vi "main.vi"() -> ()   [LabVIEW 2020]
uses:
  Desktop/eTPC/subVIs for MKS/INITIALIZATION PFEIFFER.ctl
  INITIALIZATION.ctl
  <instrlib>/PV ActiveLine/Public/Action-Status/PV ActiveLine - Sensor On-Off (TPG362).vi
  <instrlib>/PV ActiveLine/Public/Data/PV ActiveLine - Measurement Data all Gauges (TPG362).vi
  <instrlib>/PV ActiveLine/PV ActiveLine.lvlib
panel:
  in  "BACK TO CONFIG":bool
  out "CAEN":string
  out "NI DAQ":string
  out "PF":string
  out "MKS":string
  out "PF UNIT":i8 min=0 max=2
  out "PF UNIT":i8 min=0 max=2
  out "NI RELAYS STATUS":bool[](array[boolean]) caption="data"
  out "PF RESAYS STATUS":bool[](array[boolean])
  out "MKS RELAYS STATUS":bool[](array[boolean])
  out "MKS FLOW":dbl[](array[numeric])
  in  "NI OPEN VALVE":bool
  out "PF 4":bool
  out "PF 3":bool
  out "PF 2":bool
  out "PF 1":bool
  out "MKS 12":bool
  out "MKS 11":bool
  out "MKS 10":bool
  out "MKS 9":bool
  out "MKS 8":bool
  out "MKS 7":bool
  out "MKS 6":bool
  out "MKS 5":bool
  out "MKS 4":bool
  out "MKS 3":bool
  out "MKS 2":bool
  out "MKS1":bool
  out "NI 8":bool
  out "NI 7":bool
  out "NI 6":bool
  out "ALARM":bool
  out "V4":bool
  out "V3":bool
  out "V2":bool
  out "V1":bool
  in  "Tab Control":enum32{"MKS", "PFEIFEER", "CAEN", "DAQ", "LOG"}(tab)
  in  "CONNECT WITH MKS":bool
  in  "MKS":T1={"ADDRESS"="001", "BAUDE RATE"=19200, "VISA RESOURCE NAME"="", "parity (0:none)"=0} caption="Cluster 2" {"parity (0:none)" items=["None", "Odd", "Even", "Mark", "Space"]; "BAUDE RATE" items=["38400"=38400, "19200"=19200, "9600"=9600, "4800"=4800]}
  in  "MKS SET UNIT":string(combo)="MBAR" caption="MKS UNITS"
  in  "CONNECT WITH PFIFER":bool
  in  "PFEIFFER":T2={"BAUDE RATE"=enum."9600", "VISA RESOURCE NAME"=""}
  out "Device Type":string
  out "Serial Number":string
  out "Gauge out":string[](array[string])
  in  "PF SET UNIT":i8(ring) items=["mbar / bar", "Torr", "Pascal", "Micron", "hPascal (default)", "Volt"]
  in  "CONNECT WITH CAEN":bool
  in  "CAEN 2":T2={"BAUDE RATE"=enum."9600", "VISA RESOURCE NAME"=""}
  out "CAEN MODEL":string
  in  "DAQ NAME":tag="Dev3"
  in  "CONNECT WITH DAQ":bool
  in  "LOG FILE":path
  out "FILE":string
  out "status":bool
  out "code":i32
  out "FILENAME":refnum<file>
  in  "CAEN SET VOLTAGE B":bool
  in  "CAEN SET CURRENT B":bool
  out "PF Pressure CH1":dbl format="%.3e"
  out "PF Pressure CH2":dbl format="%.3e"
  out "CAEN MON CURRENT":dbl[](array[numeric])
  out "CAEN MON VOLTAGE":dbl[](array[numeric])
  in  "CAEN SET VOLTAGE":dbl
  in  "CAEN SET CURRENT":dbl
  in  "CAEN CHANNEL":string(combo)
  out "MKS PRESSURE":dbl[](array[numeric])
  out "MON ERROR":errorcluster
  in  "START":bool
  out "MKS UNIT":string
  out "INITN ERROR":errorcluster
  out "END ERROR":errorcluster
  in  "stop":bool
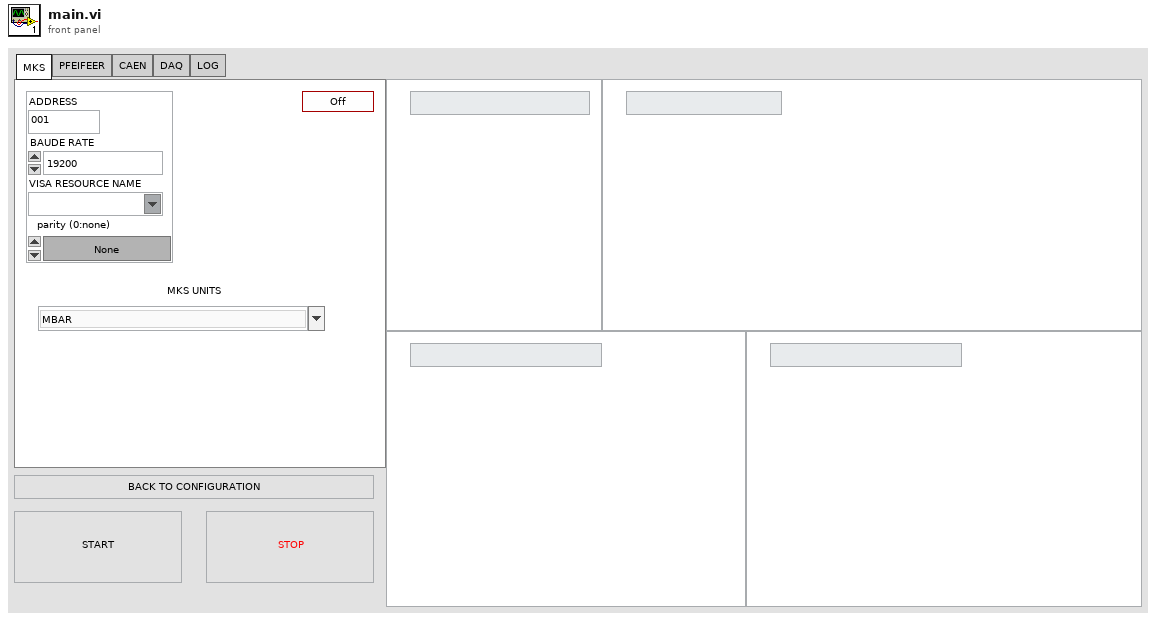
[diagram p1: front panel]
types:
  T1 = typedef "INITIALIZATION.ctl" = cluster{"ADDRESS":string, "BAUDE RATE":u32, "VISA RESOURCE NAME":refnum<visa-resource-name>, "parity (0:none)":u16}
  T2 = typedef "INITIALIZATION PFEIFFER.ctl" = cluster{"BAUDE RATE":enum32{"38400", "19200", "9600", "4800"}, "VISA RESOURCE NAME":refnum<visa-resource-name>}
  T3 = enum16{"open", "replace", "create", "open or create", "replace or create", "replace or create with confirmation"}
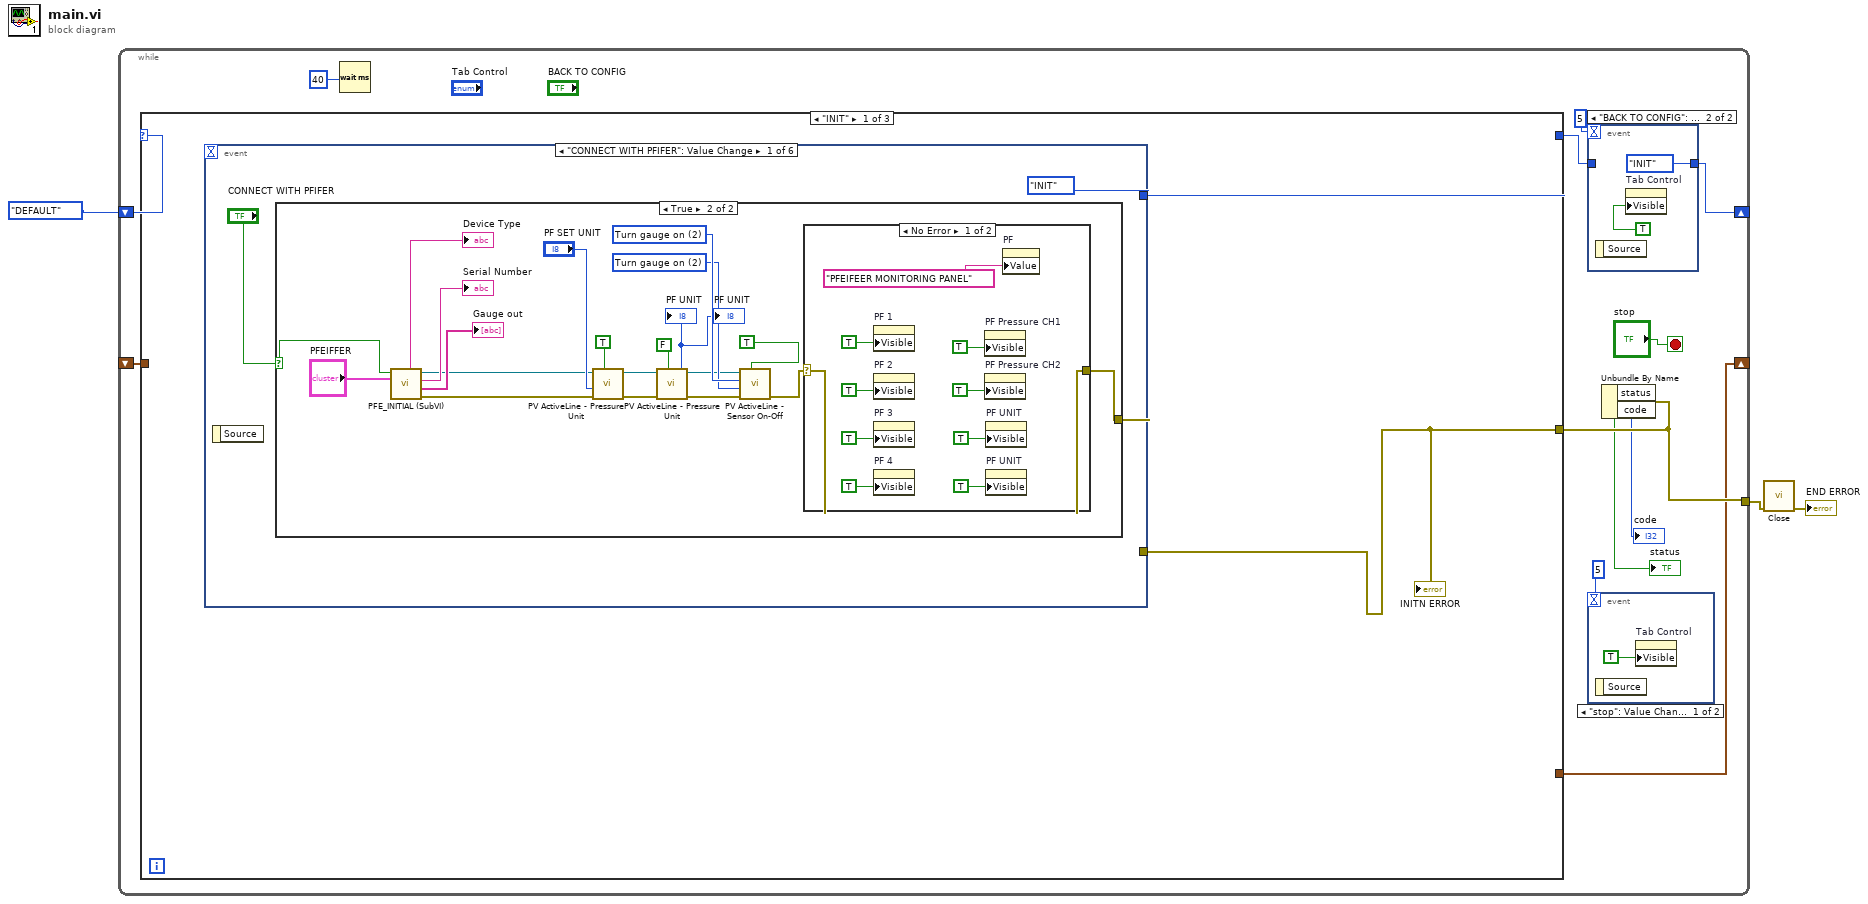
[diagram p0: block diagram]
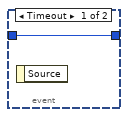
[diagram p2: hidden frame]
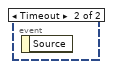
[diagram p3: hidden frame]
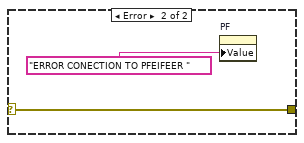
[diagram p5: hidden frame]
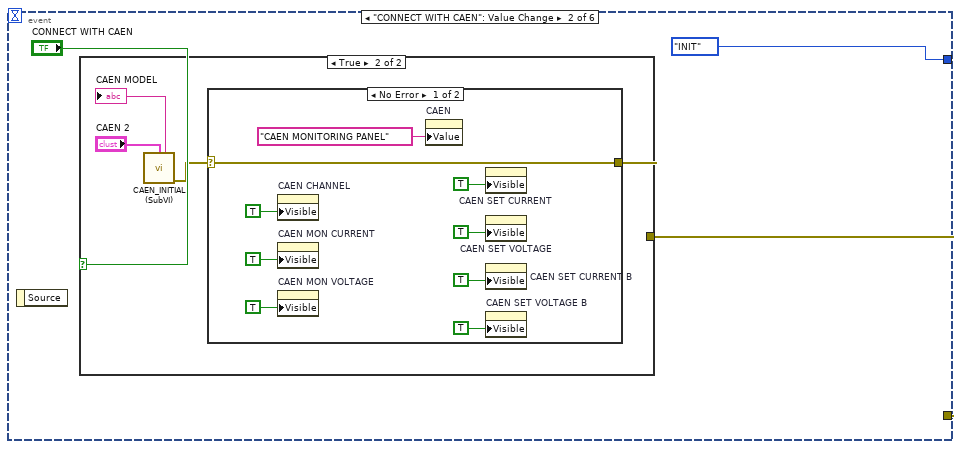
[diagram p6: hidden frame]
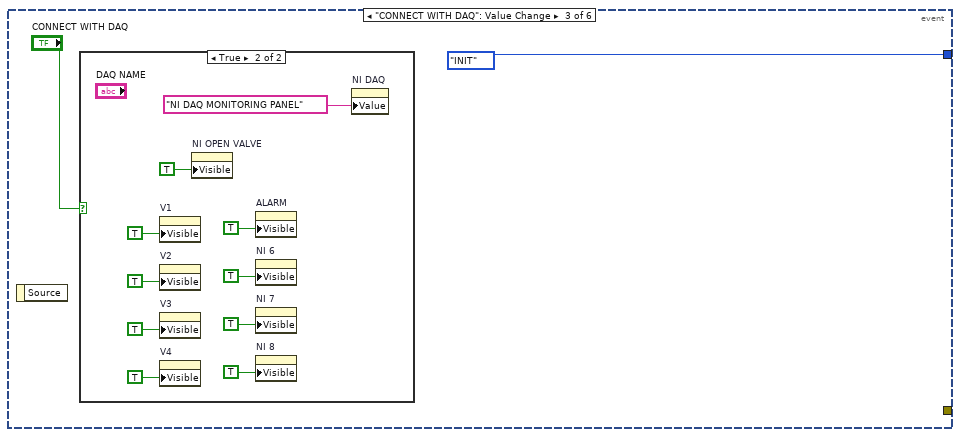
[diagram p9: hidden frame]
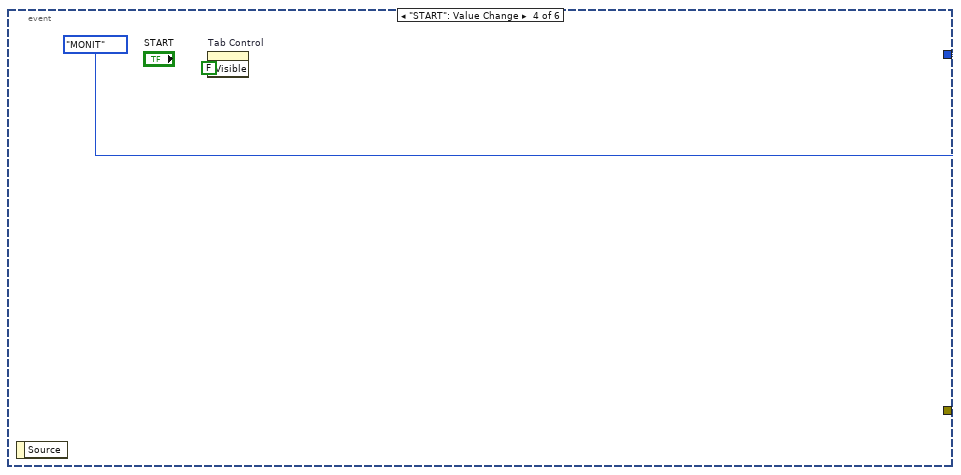
[diagram p11: hidden frame]
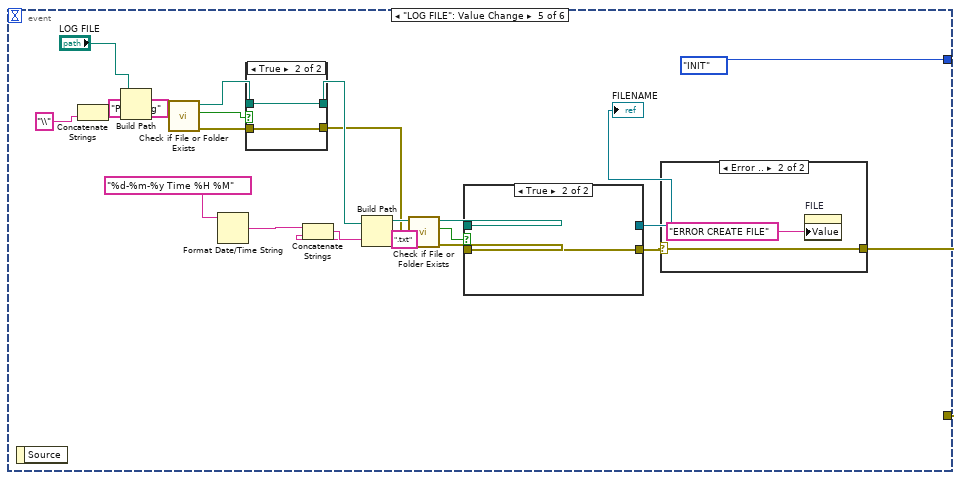
[diagram p12: hidden frame]
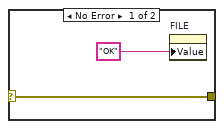
[diagram p13: hidden frame]
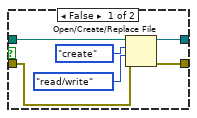
[diagram p14: hidden frame]
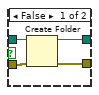
[diagram p15: hidden frame]
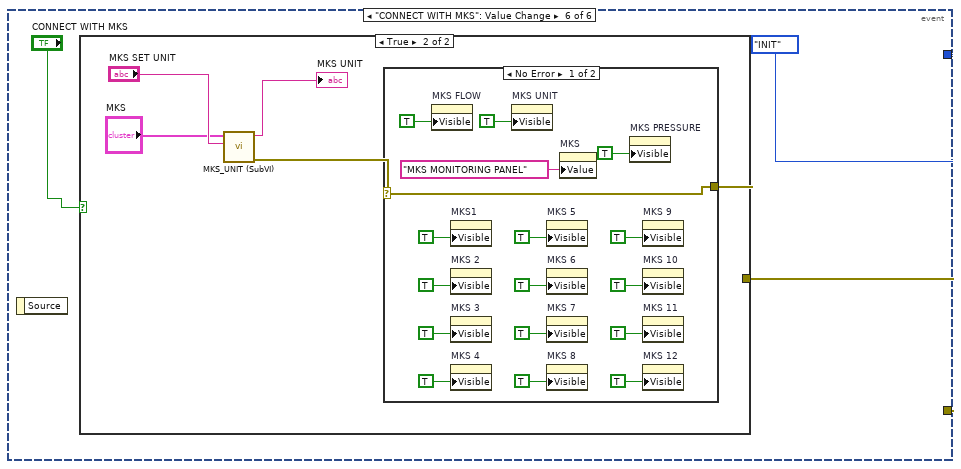
[diagram p16: hidden frame]
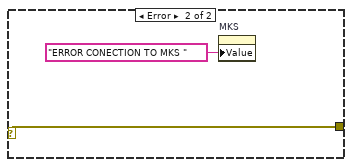
[diagram p18: hidden frame]
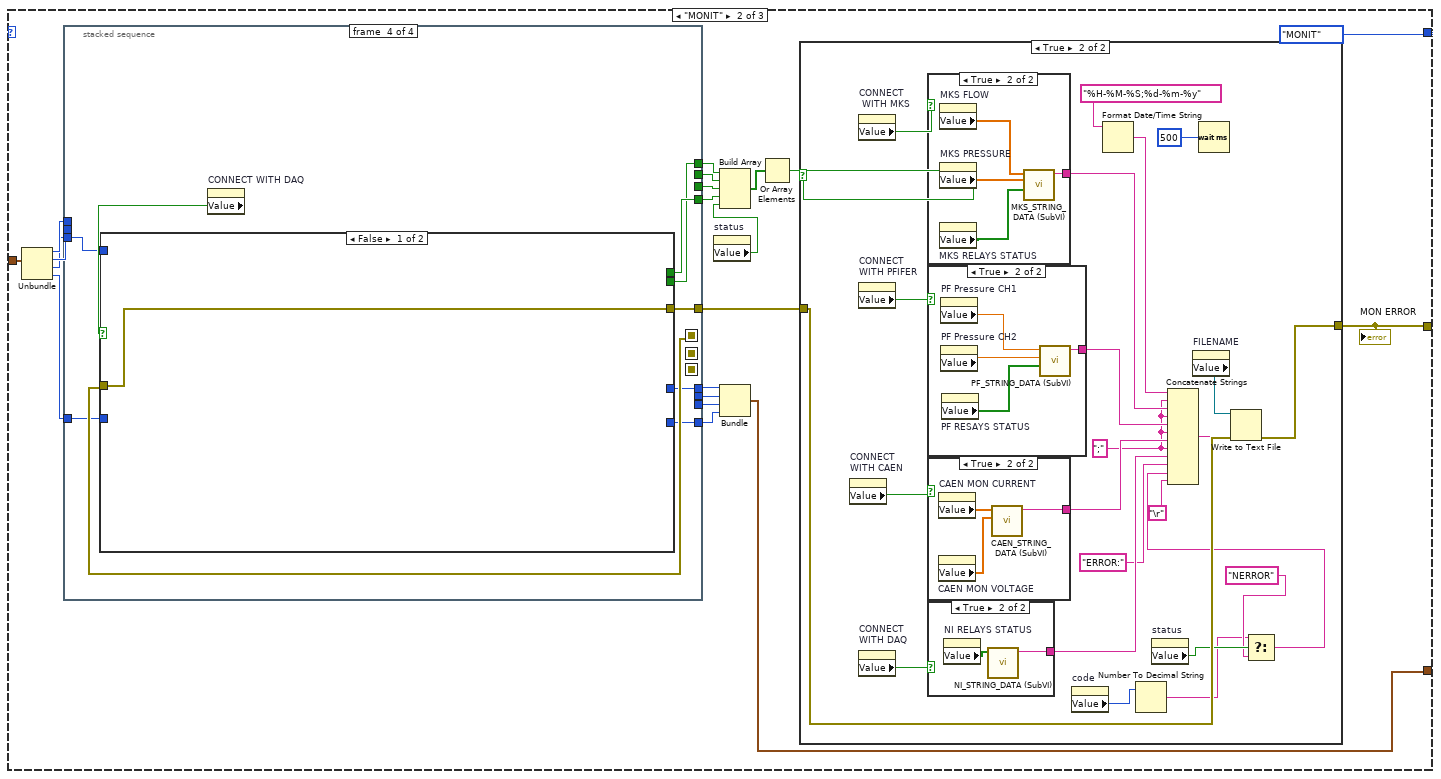
[diagram p19: hidden frame]
diagram:
  n1 = while {
    shift-right: [w4] -> _
    shift-left: enum16{"DEFAULT", "INIT", "MONIT"}."DEFAULT" ("Enum") -> [w15]
    tunnel: [w14] -> w2
    shift-right: [w11] -> _
    shift-left: _ -> [w10]
    stop <- "stop" stop-if-true
    n2 = case shown="\"INIT\"" w15 {
      tunnel: [w20 enum16{"DEFAULT", "INIT", "MONIT"}."MONIT" ("Enum") enum16{"DEFAULT", "INIT", "MONIT"}."INIT" ("Enum")] -> w8
      tunnel: [w21 w171 _] -> w14
      tunnel: [_ w157 _] -> w11
      tunnel: w10 -> [_ w166 _]
      frame "INIT" {
        n3 = event shown="[0] \"CONNECT WITH PFIFER\": Value Change" {
          selector: _ -> [_ _ _ _ _ _]
          dyn-events: _ -> [_ _ _ _ _ _]
          timeout: _ -> [_ _ _ _ _ _]
          tunnel: [w23 w57 _ _ w88 w128] -> w21
          tunnel: [enum16{"DEFAULT", "INIT", "MONIT"}."INIT" ("Enum") enum16{"DEFAULT", "INIT", "MONIT"}."INIT" ("Enum") enum16{"DEFAULT", "INIT", "MONIT"}."INIT" ("Enum") enum16{"DEFAULT", "INIT", "MONIT"}."MONIT" ("Enum") enum16{"DEFAULT", "INIT", "MONIT"}."INIT" ("Enum") enum16{"DEFAULT", "INIT", "MONIT"}."INIT" ("Enum")] -> w20
          event "CONNECT WITH PFIFER": Value Change {
            n4 = event-data() -> ()  [unwired: 1 in, 1 out]
            n5 = case shown="True" "CONNECT WITH PFIFER" {
              selector: "CONNECT WITH PFIFER" -> [_ w44]
              tunnel: [_ w25] -> w23
              frame False {
              }
              frame True {
                w35 = u8 2 items=["No status change", "Turn gauge off", "Turn gauge on"] ("Sensor 2 Set")
                w36 = u8 2 items=["No status change", "Turn gauge off", "Turn gauge on"] ("Sensor 1 Set")
                n6 = call "PFE_INITIAL (SubVI).vi"("Cluster"="PFEIFFER", "CONNECT WITH PFEIFFER"=w44) -> ("error out"=w38:errorcluster, "Gauge out"=→"Gauge out":string[], "Serial Number"=→"Serial Number":string, "Referenz out"=w39:refnum<visa-resource-name>, "Device Type"=→"Device Type":string)  [unwired: 5 in]
                n7 = call <instrlib>:"PV ActiveLine - Pressure Unit.vi"("W/R"=TRUE, "Fehler (Eingang)"=w38, "Unit Set"="PF SET UNIT", "Referenz in"=w39) -> ("Cluster (Ausgang)"=w31:errorcluster, "Referenz out"=w32:refnum<visa-resource-name>)  [unwired: 5 in, 1 out]
                n8 = call <instrlib>:"PV ActiveLine - Pressure Unit.vi"("W/R"=FALSE, "Fehler (Eingang)"=w31, "Referenz in"=w32) -> ("Cluster (Ausgang)"=w30:errorcluster, "Unit Get"=→"PF UNIT" →"PF UNIT":i8, "Referenz out"=w29:refnum<visa-resource-name>)  [unwired: 6 in]
                n9 = call-poly <instrlib>:"PV ActiveLine - Sensor On-Off.vi"("W/R"=TRUE, "Fehler (Eingang)"=w30, "Sensor 2 Set"=w35, "Sensor 1 Set"=w36, "Referenz in"=w29) -> ("Cluster (Ausgang)"=w26:errorcluster)  [unwired: 3 in, 3 out]
                n10 = case shown="No Error" w26 {
                  selector: w26 -> [w45 w56]
                  tunnel: [w45 w56] -> w25
                  frame No Error {
                    n11 = property on="PF 1" class="Bool (strict)"("Visible"=TRUE) -> ()  [unwired: 2 in, 2 out]
                    n12 = property on="PF 2" class="Bool (strict)"("Visible"=TRUE) -> ()  [unwired: 2 in, 2 out]
                    n13 = property on="PF 3" class="Bool (strict)"("Visible"=TRUE) -> ()  [unwired: 2 in, 2 out]
                    n14 = property on="PF 4" class="Bool (strict)"("Visible"=TRUE) -> ()  [unwired: 2 in, 2 out]
                    n15 = property on="PF Pressure CH1" class="DigNum (strict)"("Visible"=TRUE) -> ()  [unwired: 2 in, 2 out]
                    n16 = property on="PF Pressure CH2" class="DigNum (strict)"("Visible"=TRUE) -> ()  [unwired: 2 in, 2 out]
                    n17 = property on="PF UNIT" class="DigNum (strict)"("Visible"=TRUE) -> ()  [unwired: 2 in, 2 out]
                    n18 = property on="PF UNIT" class="DigNum (strict)"("Visible"=TRUE) -> ()  [unwired: 2 in, 2 out]
                    n19 = property on="PF" class="Str"("Value"="PFEIFEER MONITORING PANEL" ("PF")) -> ()  [unwired: 2 in, 2 out]
                  }
                  frame Error {
                    n20 = property on="PF" class="Str"("Value"="ERROR CONECTION TO PFEIFEER " ("PF")) -> ()  [unwired: 2 in, 2 out]
                  }
                }
              }
            }
          }
          event "CONNECT WITH CAEN": Value Change {
            n21 = event-data() -> ()  [unwired: 1 in, 1 out]
            n22 = case shown="True" "CONNECT WITH CAEN" {
              tunnel: [_ w61] -> w57
              frame False {
              }
              frame True {
                n23 = call "CAEN_INITIAL (SubVI).vi"("Cluster in"="CAEN 2") -> ("error out"=w63:errorcluster, "result string"=→"CAEN MODEL":string)  [unwired: 9 in]
                n24 = case shown="No Error" w63 {
                  selector: w63 -> [w64 w73]
                  tunnel: [w64 w73] -> w61
                  frame No Error {
                    n25 = property on="CAEN CHANNEL" class="CmbBox"("Visible"=TRUE) -> ()  [unwired: 2 in, 2 out]
                    n26 = property on="CAEN MON CURRENT" class="Arr (strict)"("Visible"=TRUE) -> ()  [unwired: 2 in, 2 out]
                    n27 = property on="CAEN MON VOLTAGE" class="Arr (strict)"("Visible"=TRUE) -> ()  [unwired: 2 in, 2 out]
                    n28 = property on="CAEN" class="Str"("Value"="CAEN MONITORING PANEL" ("CAEN")) -> ()  [unwired: 2 in, 2 out]
                    n29 = property on="CAEN SET CURRENT" class="DigNum (strict)"("Visible"=TRUE) -> ()  [unwired: 2 in, 2 out]
                    n30 = property on="CAEN SET VOLTAGE" class="DigNum (strict)"("Visible"=TRUE) -> ()  [unwired: 2 in, 2 out]
                    n31 = property on="CAEN SET CURRENT B" class="Bool"("Visible"=TRUE) -> ()  [unwired: 2 in, 2 out]
                    n32 = property on="CAEN SET VOLTAGE B" class="Bool"("Visible"=TRUE) -> ()  [unwired: 2 in, 2 out]
                  }
                  frame Error {
                  }
                }
              }
            }
          }
          event "CONNECT WITH DAQ": Value Change {
            n33 = event-data() -> ()  [unwired: 1 in, 1 out]
            n34 = case shown="True" "CONNECT WITH DAQ" {
              frame False {
              }
              frame True {
                n35 = property on="V1" class="Bool (strict)"("Visible"=TRUE) -> ()  [unwired: 2 in, 2 out]
                n36 = property on="V2" class="Bool (strict)"("Visible"=TRUE) -> ()  [unwired: 2 in, 2 out]
                n37 = property on="V3" class="Bool (strict)"("Visible"=TRUE) -> ()  [unwired: 2 in, 2 out]
                n38 = property on="V4" class="Bool (strict)"("Visible"=TRUE) -> ()  [unwired: 2 in, 2 out]
                n39 = property on="NI OPEN VALVE" class="Bool (strict)"("Visible"=TRUE) -> ()  [unwired: 2 in, 2 out]
                n40 = property on="ALARM" class="Bool (strict)"("Visible"=TRUE) -> ()  [unwired: 2 in, 2 out]
                n41 = property on="NI 6" class="Bool (strict)"("Visible"=TRUE) -> ()  [unwired: 2 in, 2 out]
                n42 = property on="NI 7" class="Bool (strict)"("Visible"=TRUE) -> ()  [unwired: 2 in, 2 out]
                n43 = property on="NI 8" class="Bool (strict)"("Visible"=TRUE) -> ()  [unwired: 2 in, 2 out]
                n44 = property on="NI DAQ" class="Str"("Value"="NI DAQ MONITORING PANEL" ("NI DAQ")) -> ()  [unwired: 2 in, 2 out]
              }
            }
          }
          event "START": Value Change {
            n45 = event-data() -> ()  [unwired: 1 in, 1 out]
            n46 = property on="Tab Control" class="TabCtl (strict)"("Visible"=FALSE) -> ()  [unwired: 2 in, 2 out]
          }
          event "LOG FILE": Value Change {
            n47 = event-data() -> ()  [unwired: 1 in, 1 out]
            n48 = Concatenate Strings("PPAC_log" ("String 2"), "\\" ("element")) -> (w105:string)
            n49 = Build Path(base path="LOG FILE", name or relative path=w105) -> (appended path=w109:path)
            n50 = call <vilib>:"Check if File or Folder Exists.vi"("path"=w109) -> ("error out"=w90:errorcluster, "file or folder exists?"=w107:bool, "dup path"=w108:path)  [unwired: 8 in]
            n51 = Format Date/Time String(time format string (%c)="%d-%m-%y Time %H %M") -> (date/time string=w101:string)  [unwired: 2 in]
            n52 = case shown="True" w107 {
              tunnel: w108 -> [w124 w126]
              tunnel: [w123 w126] -> w102
              tunnel: w90 -> [w122 w125]
              tunnel: [w121 w125] -> w89
              frame False {
                n53 = Create Folder(path (use dialog)=w124, error in=w122) -> (created path=w123:path, error out=w121:errorcluster)  [unwired: 1 in, 1 out]
              }
              frame True {
              }
            }
            n54 = Concatenate Strings(w101, ".txt" ("string")) -> (w100:string)
            n55 = Build Path(base path=w102, name or relative path=w100) -> (appended path=w98:path)
            n56 = call <vilib>:"Check if File or Folder Exists.vi"("error in (no error)"=w89, "path"=w98) -> ("error out"=w91:errorcluster, "file or folder exists?"=w95:bool, "dup path"=w97:path)  [unwired: 7 in]
            n57 = case shown="True" w95 {
              tunnel: w97 -> [w117 _]
              tunnel: [w116 _] -> w93
              tunnel: [w115 w120] -> w92
              tunnel: w91 -> [w114 w120]
              frame False {
                n58 = Open/Create/Replace File(file path (use dialog)=w117, error in=w114, operation (0:open)=T3."create", access (0:read/write)=enum16{"read/write", "read-only", "write-only"}."read/write") -> (refnum out=w116:refnum<file>, error out=w115:errorcluster)  [unwired: 2 in, 1 out]
              }
              frame True {
              }
            }
            "FILENAME" <- w93
            n59 = case shown="Error .." w92 {
              selector: w92 -> [w111 w113]
              tunnel: [w111 w113] -> w88
              frame No Error {
                n60 = property on="FILE" class="Str"("Value"="OK" ("FILE")) -> ()  [unwired: 2 in, 2 out]
              }
              frame Error {
                n61 = property on="FILE" class="Str"("Value"="ERROR CREATE FILE" ("FILE")) -> ()  [unwired: 2 in, 2 out]
              }
            }
          }
          event "CONNECT WITH MKS": Value Change {
            n62 = event-data() -> ()  [unwired: 1 in, 1 out]
            n63 = case shown="True" "CONNECT WITH MKS" {
              tunnel: [_ w130] -> w128
              frame False {
              }
              frame True {
                n64 = call "MKS_UNIT (SubVI).vi"("MKS UNITS"="MKS SET UNIT", "Cluster in"="MKS") -> ("error out"=w131:errorcluster, "result string"=→"MKS UNIT":string)  [unwired: 8 in]
                n65 = case shown="No Error" w131 {
                  selector: w131 -> [w135 w153]
                  tunnel: [w135 w153] -> w130
                  frame No Error {
                    n66 = property on="MKS FLOW" class="Arr (strict)"("Visible"=TRUE) -> ()  [unwired: 2 in, 2 out]
                    n67 = property on="MKS1" class="Bool (strict)"("Visible"=TRUE) -> ()  [unwired: 2 in, 2 out]
                    n68 = property on="MKS 2" class="Bool (strict)"("Visible"=TRUE) -> ()  [unwired: 2 in, 2 out]
                    n69 = property on="MKS 3" class="Bool (strict)"("Visible"=TRUE) -> ()  [unwired: 2 in, 2 out]
                    n70 = property on="MKS 4" class="Bool (strict)"("Visible"=TRUE) -> ()  [unwired: 2 in, 2 out]
                    n71 = property on="MKS UNIT" class="Str"("Visible"=TRUE) -> ()  [unwired: 2 in, 2 out]
                    n72 = property on="MKS 5" class="Bool (strict)"("Visible"=TRUE) -> ()  [unwired: 2 in, 2 out]
                    n73 = property on="MKS 6" class="Bool (strict)"("Visible"=TRUE) -> ()  [unwired: 2 in, 2 out]
                    n74 = property on="MKS 7" class="Bool (strict)"("Visible"=TRUE) -> ()  [unwired: 2 in, 2 out]
                    n75 = property on="MKS 8" class="Bool (strict)"("Visible"=TRUE) -> ()  [unwired: 2 in, 2 out]
                    n76 = property on="MKS" class="Str"("Value"="MKS MONITORING PANEL" ("String")) -> ()  [unwired: 2 in, 2 out]
                    n77 = property on="MKS PRESSURE" class="Arr (strict)"("Visible"=TRUE) -> ()  [unwired: 2 in, 2 out]
                    n78 = property on="MKS 9" class="Bool (strict)"("Visible"=TRUE) -> ()  [unwired: 2 in, 2 out]
                    n79 = property on="MKS 10" class="Bool (strict)"("Visible"=TRUE) -> ()  [unwired: 2 in, 2 out]
                    n80 = property on="MKS 11" class="Bool (strict)"("Visible"=TRUE) -> ()  [unwired: 2 in, 2 out]
                    n81 = property on="MKS 12" class="Bool (strict)"("Visible"=TRUE) -> ()  [unwired: 2 in, 2 out]
                  }
                  frame Error {
                    n82 = property on="MKS" class="Str"("Value"="ERROR CONECTION TO MKS " ("String")) -> ()  [unwired: 2 in, 2 out]
                  }
                }
              }
            }
          }
        }
        "INITN ERROR" <- w21
      }
      frame "MONIT" {
        n83 = Unbundle(w166) -> (w165:u32, w162:u32, w161:u32, w155:i16)
        n84 = stacked-sequence {
          seq-local: [w218 _ _ _] -> [_ w243 _ _]
          seq-local: [_ w244 _ _] -> [_ _ w269 _]
          seq-local: [_ _ w270 _] -> [_ _ _ w296]
          tunnel: [_ _ _ w295] -> w172
          tunnel: [_ _ _ w294] -> w168
          tunnel: [_ _ w268 _] -> w167
          tunnel: [w217 _ _ _] -> w158
          tunnel: w165 -> [w216 _ _ _]
          tunnel: [w215 _ _ _] -> w164
          tunnel: [_ _ w267 _] -> w163
          tunnel: w162 -> [_ _ w266 _]
          tunnel: w161 -> [_ _ _ w293]
          tunnel: [_ _ _ w292] -> w160
          tunnel: [_ _ _ w291] -> w156
          tunnel: w155 -> [_ _ _ w290]
          tunnel: [_ _ _ w289] -> w154
          frame #0 {
            n85 = property on="CONNECT WITH MKS" class="Bool (strict)"() -> ("Value"=w219:bool)  [unwired: 2 in, 2 out]
            n86 = case shown="True" w219 {
              tunnel: [_ w241] -> w218
              tunnel: [_ w221] -> w217
              tunnel: w216 -> [_ w222]
              tunnel: [_ w220] -> w215
              frame False {
              }
              frame True {
                n87 = property on="MKS" class="Clust (strict)"() -> ("Value"=w239:T1)  [unwired: 2 in, 2 out]
                n88 = call "MKS_FLOW (SubVI).vi"("Cluster in"=w239) -> ("error out"=w237:errorcluster, "DBL out"=→"MKS FLOW":dbl[])  [unwired: 9 in]
                n89 = call "MKS_PRESSURE (SubVI).vi"("error in (no error)"=w237, "Cluster in"=w239) -> ("error out"=w238:errorcluster, "DBL out"=→"MKS PRESSURE":dbl[])  [unwired: 8 in]
                n90 = call "MKS_RELAYS (SubVI).vi"("error in (no error)"=w238, "Cluster in"=w239) -> ("error out"=w241:errorcluster, "x != 0?"=w223:bool[])  [unwired: 8 in]
                "MKS RELAYS STATUS" <- w223
                n91 = Index Array(array=w223) -> (element #1=→"MKS1":bool, element #2=→"MKS 2":bool, element #3=→"MKS 3":bool, element #4=→"MKS 4":bool, element #5=→"MKS 5":bool, element #6=→"MKS 6":bool, element #7=→"MKS 7":bool, element #8=→"MKS 8":bool, element #9=→"MKS 9":bool, element #10=→"MKS 10":bool, element #11=→"MKS 11":bool, element #12=→"MKS 12":bool)  [unwired: 12 in]
                n92 = Boolean Array To Number(Boolean array=w223) -> (number=w221:u32)
                n93 = Not Equal?(x=w222, y=w221) -> (x != y?=w220:bool)
              }
            }
          }
          frame #1 {
            n94 = property on="CONNECT WITH CAEN" class="Bool (strict)"() -> ("Value"=w242:bool)  [unwired: 2 in, 2 out]
            n95 = case shown="True" w242 {
              tunnel: w243 -> [w245 w249]
              tunnel: [w245 w247] -> w244
              frame False {
              }
              frame True {
                n96 = property on="CAEN 2" class="Clust (strict)"() -> ("Value"=w246:T2)  [unwired: 2 in, 2 out]
                n97 = event shown="[2] \"CAEN SET VOLTAGE B\": Value Change" {
                  selector: _ -> [_ _ _]
                  dyn-events: _ -> [_ _ _]
                  timeout: 20 -> [_ _ _]
                  tunnel: "CAEN CHANNEL" -> [w259 _ w264]
                  tunnel: w246 -> [w255 _ w262]
                  tunnel: [w258 w260 w261] -> w248
                  tunnel: w249 -> [w256 w260 w263]
                  event "CAEN SET CURRENT B": Value Change {
                    n98 = event-data() -> ()  [unwired: 1 in, 1 out]
                    n99 = call "CAEN_CUR_SET (SubVI).vi"("Numeric"="CAEN SET CURRENT", "error in (no error)"=w256, "CHANNEL"=w259, "Cluster in 2"=w255) -> ("error out"=w258:errorcluster)  [unwired: 7 in]
                  }
                  event Timeout {
                    n100 = event-data() -> ()  [unwired: 1 in, 1 out]
                  }
                  event "CAEN SET VOLTAGE B": Value Change {
                    n101 = event-data() -> ()  [unwired: 1 in, 1 out]
                    n102 = call "CAEN_VOL_SET (SubVI).vi"("Numeric"="CAEN SET VOLTAGE", "error in (no error)"=w263, "CHANNEL"=w264, "Cluster in 2"=w262) -> ("error out"=w261:errorcluster)  [unwired: 7 in]
                  }
                }
                n103 = call "CAEN_CUR_MON (SubVI).vi"("error in (no error)"=w248, "Cluster in"=w246) -> ("error out"=w254:errorcluster, "DBL out"=→"CAEN MON CURRENT":dbl[])  [unwired: 8 in]
                n104 = call "CAEN_VOL_MON (SubVI).vi"("error in (no error)"=w254, "Cluster in 2"=w246) -> ("error out"=w247:errorcluster, "DBL out"=→"CAEN MON VOLTAGE":dbl[])  [unwired: 8 in]
              }
            }
          }
          frame #2 {
            n105 = property on="CONNECT WITH PFIFER" class="Bool (strict)"() -> ("Value"=w271:bool)  [unwired: 2 in, 2 out]
            n106 = case shown="True" w271 {
              tunnel: w269 -> [w272 w284]
              tunnel: [w272 w283] -> w270
              tunnel: [_ w275] -> w267
              tunnel: [_ w273] -> w268
              tunnel: w266 -> [_ w274]
              frame False {
              }
              frame True {
                n107 = property on="PFEIFFER" class="Clust (strict)"() -> ("Value"=w281:T2)  [unwired: 2 in, 2 out]
                n108 = Unbundle By Name(w281) -> ("VISA RESOURCE NAME"=w282:refnum<visa-resource-name>)
                n109 = call-poly <instrlib>:"PV ActiveLine - Measurement Data all Gauges.vi"("Fehler (Eingang)"=w284, "Referenz in"=w282) -> ("Cluster (Ausgang)"=w286:errorcluster, "Pressure CH2"=→"PF Pressure CH2":dbl, "Pressure CH1"=→"PF Pressure CH1":dbl, "Referenz out"=w285:refnum<visa-resource-name>)  [unwired: 4 in, 2 out]
                n110 = call <instrlib>:"PV ActiveLine - SwitchingFunctionStatus.vi"("Referenz in"=w285, "Fehler (Eingang)"=w286) -> ("x != 0?"=w280:bool[], "Cluster (Ausgang)"=w283:errorcluster)  [unwired: 15 in, 1 out]
                "PF RESAYS STATUS" <- w280
                n111 = Index Array(array=w280) -> (element #1=→"PF 1":bool, element #2=→"PF 2":bool, element #3=→"PF 3":bool, element #4=→"PF 4":bool)  [unwired: 4 in]
                n112 = Boolean Array To Number(Boolean array=w280) -> (number=w273:u32)
                n113 = Not Equal?(x=w274, y=w273) -> (x != y?=w275:bool)
              }
            }
          }
          frame #3 {
            n114 = property on="CONNECT WITH DAQ" class="Bool (strict)"() -> ("Value"=w297:bool)  [unwired: 2 in, 2 out]
            n115 = case shown="False" w297 {
              tunnel: [w298 w316] -> w295
              tunnel: w296 -> [w298 w315]
              tunnel: [_ w304] -> w294
              tunnel: w293 -> [_ w305]
              tunnel: [_ w303] -> w292
              tunnel: [_ w301] -> w291
              tunnel: w290 -> [_ w300]
              tunnel: [_ w299] -> w289
              frame False {
              }
              frame True {
                n116 = property on="DAQ NAME" class="DAQmxName"() -> ("Value"=w318:string)  [unwired: 2 in, 2 out]
                n117 = Boolean To (0,1)(Boolean="NI OPEN VALVE") -> (0, 1=w301:i16)
                n118 = Build Array("NI OPEN VALVE") -> (w319:bool[])
                n119 = Not Equal?(x=w301, y=w300) -> (x != y?=w299:bool)
                n120 = call "SEND DATA"("data"=w319, "error in"=w315, "device name"=w318) -> ("error out"=w317:errorcluster)  [unwired: 15 in, 1 out]
                n121 = call "RECIVE DATA"("error in"=w317, "device name"=w318) -> ("data"=w314:bool[], "error out"=w316:errorcluster)  [unwired: 15 in, 1 out]
                "NI RELAYS STATUS" <- w314
                n122 = Index Array(array=w314) -> (element #1=→"V1":bool, element #2=→"V2":bool, element #3=→"V3":bool, element #4=→"V4":bool, element #5=→"ALARM":bool, element #6=→"NI 6":bool, element #7=→"NI 7":bool, element #8=→"NI 8":bool)  [unwired: 8 in]
                n123 = Boolean Array To Number(Boolean array=w314) -> (number=w304:u32)
                n124 = Not Equal?(x=w305, y=w304) -> (x != y?=w303:bool)
              }
            }
          }
        }
        n125 = property on="status" class="Bool (strict)"() -> ("Value"=w159:bool)  [unwired: 2 in, 2 out]
        n126 = Build Array(w154, w164, w163, w160, w159) -> (w170:bool[])
        n127 = Bundle(w158, w167, w168, w156) -> (w157:cluster{u32, u32, u32, i16})  [unwired: 1 in]
        n128 = Or Array Elements(Boolean array=w170) -> (logical OR=w169:bool)
        n129 = case shown="True" w169 {
          tunnel: w172 -> [w174 w197]
          tunnel: [w174 w196] -> w171
          frame False {
          }
          frame True {
            w183 = ";" ("string")
            n130 = property on="CONNECT \nWITH CAEN" class="Bool (strict)"() -> ("Value"=w175:bool)  [unwired: 2 in, 2 out]
            n131 = property on="CONNECT\n WITH MKS" class="Bool (strict)"() -> ("Value"=w191:bool)  [unwired: 2 in, 2 out]
            n132 = property on="CONNECT \nWITH PFIFER" class="Bool (strict)"() -> ("Value"=w192:bool)  [unwired: 2 in, 2 out]
            n133 = property on="CONNECT\nWITH DAQ" class="Bool (strict)"() -> ("Value"=w193:bool)  [unwired: 2 in, 2 out]
            n134 = case shown="True" w191 {
              tunnel: ["NCON" w213] -> w189
              frame False {
              }
              frame True {
                n135 = property on="MKS FLOW" class="Arr (strict)"() -> ("Value"=w211:dbl[])  [unwired: 2 in, 2 out]
                n136 = property on="MKS PRESSURE" class="Arr (strict)"() -> ("Value"=w214:dbl[])  [unwired: 2 in, 2 out]
                n137 = property on="MKS RELAYS STATUS" class="Arr (strict)"() -> ("Value"=w212:bool[])  [unwired: 2 in, 2 out]
                n138 = call "MKS_STRING_DATA (SubVI).vi"("Value"=w212, "Value 2"=w214, "Value 3"=w211) -> ("String"=w213:string)  [unwired: 8 in]
              }
            }
            n139 = case shown="True" w192 {
              tunnel: ["NCON" w207] -> w188
              frame False {
              }
              frame True {
                n140 = property on="PF Pressure CH1" class="DigNum (strict)"() -> ("Value"=w209:dbl)  [unwired: 2 in, 2 out]
                n141 = property on="PF Pressure CH2" class="DigNum (strict)"() -> ("Value"=w208:dbl)  [unwired: 2 in, 2 out]
                n142 = property on="PF RESAYS STATUS" class="Arr (strict)"() -> ("Value"=w206:bool[])  [unwired: 2 in, 2 out]
                n143 = call "PF_STRING_DATA (SubVI).vi"("Value"=w206, "Value 2"=w208, "Value 3"=w209) -> ("String"=w207:string)  [unwired: 8 in]
              }
            }
            n144 = case shown="True" w175 {
              tunnel: ["NCON" w202] -> w187
              frame False {
              }
              frame True {
                n145 = property on="CAEN MON CURRENT" class="Arr (strict)"() -> ("Value"=w204:dbl[])  [unwired: 2 in, 2 out]
                n146 = property on="CAEN MON VOLTAGE" class="Arr (strict)"() -> ("Value"=w203:dbl[])  [unwired: 2 in, 2 out]
                n147 = call "CAEN_STRING_DATA (SubVI).vi"("Value"=w203, "Value 2"=w204) -> ("String"=w202:string)  [unwired: 9 in]
              }
            }
            n148 = case shown="True" w193 {
              tunnel: ["NCON" w200] -> w186
              frame False {
              }
              frame True {
                n149 = property on="NI RELAYS STATUS" class="Arr (strict)"() -> ("Value"=w199:bool[])  [unwired: 2 in, 2 out]
                n150 = call "NI_STRING_DATA (SubVI).vi"("Value"=w199) -> ("String"=w200:string)  [unwired: 10 in]
              }
            }
            n151 = property on="code" class="DigNum (strict)"() -> ("Value"=w177:i32)  [unwired: 2 in, 2 out]
            n152 = Format Date/Time String(time format string (%c)="%H-%M-%S;%d-%m-%y") -> (date/time string=w190:string)  [unwired: 2 in]
            n153 = Number To Decimal String(number=w177) -> (decimal integer string=w176:string)  [unwired: 1 in]
            n154 = property on="status" class="Bool (strict)"() -> ("Value"=w179:bool)  [unwired: 2 in, 2 out]
            n155 = property on="FILENAME" class="Ref (strict)"() -> ("Value"=w195:refnum<file>)  [unwired: 2 in, 2 out]
            n156 = Wait (ms)(milliseconds to wait=u32 500) -> ()  [unwired: 1 out]
            n157 = Select(t=w176, s=w179, f="NERROR" ("string")) -> (s? t:f=w180:string)
            n158 = Concatenate Strings(w190, w183, w189, w183, w188, w183, w187, w183, w186, "ERROR:" ("string"), w180, "\r") -> (w185:string)
            n159 = Write to Text File(file (use dialog)=w195, text=w185, error in=w197) -> (error out=w196:errorcluster)  [unwired: 1 in, 2 out]
          }
        }
        "MON ERROR" <- w171
      }
      frame "DEFAULT", Default {
        n160 = property on="CONNECT WITH MKS" class="Bool (strict)"("Value"=FALSE ("CONNECT WITH MKS")) -> ()  [unwired: 2 in, 2 out]
        n161 = property on="CONNECT WITH PFIFER" class="Bool (strict)"("Value"=FALSE ("CONNECT WITH PFIFER")) -> ()  [unwired: 2 in, 2 out]
        n162 = property on="CONNECT WITH DAQ" class="Bool (strict)"("Value"=FALSE ("CONNECT WITH DAQ")) -> ()  [unwired: 2 in, 2 out]
        n163 = property on="CONNECT WITH CAEN" class="Bool (strict)"("Value"=FALSE ("CONNECT WITH CAEN")) -> ()  [unwired: 2 in, 2 out]
        n164 = property on="NI OPEN VALVE" class="Bool (strict)"("Value"=FALSE ("OPEN VALVE")) -> ()  [unwired: 2 in, 2 out]
        n165 = property on="Tab Control" class="TabCtl (strict)"("Visible"=TRUE) -> ()  [unwired: 2 in, 2 out]
        n166 = property on="CAEN SET CURRENT B" class="Bool"("Visible"=FALSE) -> ()  [unwired: 2 in, 2 out]
        n167 = property on="CAEN CHANNEL" class="CmbBox"("Visible"=FALSE) -> ()  [unwired: 2 in, 2 out]
        n168 = property on="CAEN MON CURRENT" class="Arr (strict)"("Visible"=FALSE) -> ()  [unwired: 2 in, 2 out]
        n169 = property on="CAEN MON VOLTAGE" class="Arr (strict)"("Visible"=FALSE) -> ()  [unwired: 2 in, 2 out]
        n170 = property on="CAEN SET VOLTAGE" class="DigNum (strict)"("Visible"=FALSE) -> ()  [unwired: 2 in, 2 out]
        n171 = property on="CAEN SET CURRENT" class="DigNum (strict)"("Visible"=FALSE) -> ()  [unwired: 2 in, 2 out]
        n172 = property on="CAEN SET VOLTAGE B" class="Bool"("Visible"=FALSE) -> ()  [unwired: 2 in, 2 out]
        n173 = property on="PF UNIT" class="DigNum (strict)"("Visible"=FALSE) -> ()  [unwired: 2 in, 2 out]
        n174 = property on="PF Pressure CH1" class="DigNum (strict)"("Visible"=FALSE) -> ()  [unwired: 2 in, 2 out]
        n175 = property on="PF RESAYS STATUS" class="Arr (strict)"("Visible"=FALSE) -> ()  [unwired: 2 in, 2 out]
        n176 = property on="PF Pressure CH2" class="DigNum (strict)"("Visible"=FALSE) -> ()  [unwired: 2 in, 2 out]
        n177 = property on="PF UNIT" class="DigNum (strict)"("Visible"=FALSE) -> ()  [unwired: 2 in, 2 out]
        n178 = property on="PF 1" class="Bool (strict)"("Visible"=FALSE) -> ()  [unwired: 2 in, 2 out]
        n179 = property on="PF 2" class="Bool (strict)"("Visible"=FALSE) -> ()  [unwired: 2 in, 2 out]
        n180 = property on="PF 3" class="Bool (strict)"("Visible"=FALSE) -> ()  [unwired: 2 in, 2 out]
        n181 = property on="PF 4" class="Bool (strict)"("Visible"=FALSE) -> ()  [unwired: 2 in, 2 out]
        n182 = property on="MKS1" class="Bool (strict)"("Visible"=FALSE) -> ()  [unwired: 2 in, 2 out]
        n183 = property on="MKS 5" class="Bool (strict)"("Visible"=FALSE) -> ()  [unwired: 2 in, 2 out]
        n184 = property on="MKS UNIT" class="Str"("Visible"=FALSE) -> ()  [unwired: 2 in, 2 out]
        n185 = property on="MKS FLOW" class="Arr (strict)"("Visible"=FALSE) -> ()  [unwired: 2 in, 2 out]
        n186 = property on="MKS RELAYS STATUS" class="Arr (strict)"("Visible"=FALSE) -> ()  [unwired: 2 in, 2 out]
        n187 = property on="MKS PRESSURE" class="Arr (strict)"("Visible"=FALSE) -> ()  [unwired: 2 in, 2 out]
        n188 = property on="MKS 2" class="Bool (strict)"("Visible"=FALSE) -> ()  [unwired: 2 in, 2 out]
        n189 = property on="MKS 3" class="Bool (strict)"("Visible"=FALSE) -> ()  [unwired: 2 in, 2 out]
        n190 = property on="MKS 4" class="Bool (strict)"("Visible"=FALSE) -> ()  [unwired: 2 in, 2 out]
        n191 = property on="MKS 9" class="Bool (strict)"("Visible"=FALSE) -> ()  [unwired: 2 in, 2 out]
        n192 = property on="MKS 6" class="Bool (strict)"("Visible"=FALSE) -> ()  [unwired: 2 in, 2 out]
        n193 = property on="MKS 7" class="Bool (strict)"("Visible"=FALSE) -> ()  [unwired: 2 in, 2 out]
        n194 = property on="MKS 8" class="Bool (strict)"("Visible"=FALSE) -> ()  [unwired: 2 in, 2 out]
        n195 = property on="MKS 10" class="Bool (strict)"("Visible"=FALSE) -> ()  [unwired: 2 in, 2 out]
        n196 = property on="MKS 11" class="Bool (strict)"("Visible"=FALSE) -> ()  [unwired: 2 in, 2 out]
        n197 = property on="MKS 12" class="Bool (strict)"("Visible"=FALSE) -> ()  [unwired: 2 in, 2 out]
        n198 = property on="V3" class="Bool (strict)"("Visible"=FALSE) -> ()  [unwired: 2 in, 2 out]
        n199 = property on="V4" class="Bool (strict)"("Visible"=FALSE) -> ()  [unwired: 2 in, 2 out]
        n200 = property on="ALARM" class="Bool (strict)"("Visible"=FALSE) -> ()  [unwired: 2 in, 2 out]
        n201 = property on="NI 6" class="Bool (strict)"("Visible"=FALSE) -> ()  [unwired: 2 in, 2 out]
        n202 = property on="NI 7" class="Bool (strict)"("Visible"=FALSE) -> ()  [unwired: 2 in, 2 out]
        n203 = property on="NI 8" class="Bool (strict)"("Visible"=FALSE) -> ()  [unwired: 2 in, 2 out]
        n204 = property on="V2" class="Bool (strict)"("Visible"=FALSE) -> ()  [unwired: 2 in, 2 out]
        n205 = property on="V1" class="Bool (strict)"("Visible"=FALSE) -> ()  [unwired: 2 in, 2 out]
        n206 = property on="NI OPEN VALVE" class="Bool (strict)"("Visible"=FALSE) -> ()  [unwired: 2 in, 2 out]
        n207 = property on="NI RELAYS STATUS" class="Arr (strict)"("Visible"=FALSE) -> ()  [unwired: 2 in, 2 out]
        "MKS" <- "MKS NO CONNECTED" ("String")
        "CAEN" <- "CAEN NO CONNECTED" ("String 4")
        "NI DAQ" <- "NI DAQ NO CONNECTED" ("String 3")
        "PF" <- "PF NO CONNECTED" ("String 2")
        "FILE" <- "SELECT PATH" ("FILE")
      }
    }
    n208 = Wait (ms)(milliseconds to wait=u32 40) -> ()  [unwired: 1 out]
    n209 = event shown="[1] \"BACK TO CONFIG\": Value Change" {
      selector: _ -> [_ _]
      dyn-events: _ -> [_ _]
      timeout: 5 -> [_ _]
      tunnel: w8 -> [w16 _]
      tunnel: [w16 enum16{"DEFAULT", "INIT", "MONIT"}."INIT" ("Enum")] -> w4
      event Timeout {
        n210 = event-data() -> ()  [unwired: 1 in, 1 out]
      }
      event "BACK TO CONFIG": Value Change {
        n211 = event-data() -> ()  [unwired: 1 in, 1 out]
        n212 = property on="Tab Control" class="TabCtl (strict)"("Visible"=TRUE) -> ()  [unwired: 2 in, 2 out]
      }
    }
    n213 = event shown="[0] \"stop\": Value Change" {
      selector: _ -> [_ _]
      dyn-events: _ -> [_ _]
      timeout: 5 -> [_ _]
      event "stop": Value Change {
        n214 = event-data() -> ()  [unwired: 1 in, 1 out]
        n215 = property on="Tab Control" class="TabCtl (strict)"("Visible"=TRUE) -> ()  [unwired: 2 in, 2 out]
      }
      event Timeout {
        n216 = event-data() -> ()  [unwired: 1 in, 1 out]
      }
    }
    n217 = Unbundle By Name(w14) -> ("status"=→"status":bool, "code"=→"code":i32)
  }
  n218 = call <instrlib>:"Close.vi"("error in (no error)"=w2) -> ("error out"=→"END ERROR":errorcluster)  [unwired: 10 in]
